vi "Hybrid Get Control Comp.vi"() -> (0 "Client 2":string[](array[string]))   [LabVIEW 2020]
panel:
  in  "OK Button":bool
  in  "Client":string
  # "Enter Controling Computer Name (ie Data4Mac)"
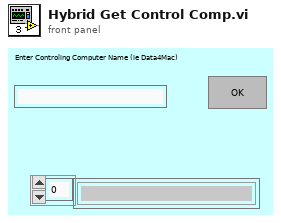
[diagram p1: front panel]
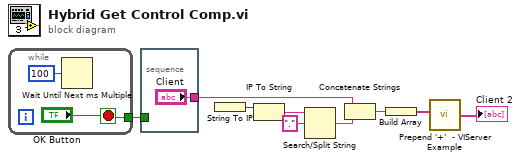
[diagram p0: block diagram]
diagram:
  n1 = while {
    tunnel: ["OK Button"] -> w9
    stop <- "OK Button" stop-if-true
    n2 = Wait Until Next ms Multiple(millisecond multiple=u32 100) -> ()  [unwired: 1 out]
  }
  n3 = stacked-sequence {
    tunnel: ["Client"] -> w4
    tunnel: w9 -> [_]
    frame #0 {
    }
  }
  n4 = String To IP() -> (0:w8:u32)  [unwired: 1 in]
  n5 = IP To String(2:w8) -> (0:w7:string)  [unwired: 1 in]
  n6 = Search/Split String(string=w7, search string/char (-)="." ("search char (-)")) -> (match + rest of string=w5:string)  [unwired: 1 in, 2 out]
  n7 = Concatenate Strings(w4, w5) -> (w3:string)
  n8 = Build Array(w3) -> (w2:string[])
  n9 = call "Prepend '+'  - VIServer Example.vi"("list in"=w2) -> ("list out"=→"Client 2":string[])
